vi "LEP_RV_ParseSerialTextOutput.vi"(7 "Serial text":string) -> (1 "Execution time":string, 2 "Stack high water mark":string, 3 "Heap high water mark":string)   [LabVIEW 2011]
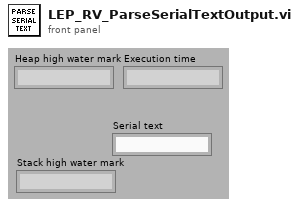
[diagram p1: front panel]
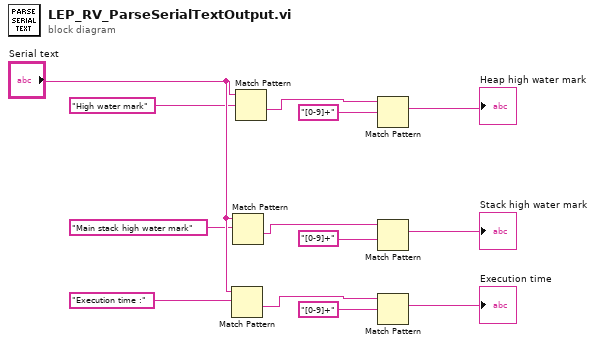
[diagram p0: block diagram]
diagram:
  n1 = Match Pattern(string="Serial text", regular expression="Execution time :") -> (after substring=w3:string)  [unwired: 1 in, 3 out]
  n2 = Match Pattern(string="Serial text", regular expression="Main stack high water mark") -> (after substring=w5:string)  [unwired: 1 in, 3 out]
  n3 = Match Pattern(string="Serial text", regular expression="High water mark") -> (after substring=w4:string)  [unwired: 1 in, 3 out]
  n4 = Match Pattern(string=w4, regular expression="[0-9]+") -> (match substring=→"Heap high water mark":string)  [unwired: 1 in, 3 out]
  n5 = Match Pattern(string=w5, regular expression="[0-9]+") -> (match substring=→"Stack high water mark":string)  [unwired: 1 in, 3 out]
  n6 = Match Pattern(string=w3, regular expression="[0-9]+") -> (match substring=→"Execution time":string)  [unwired: 1 in, 3 out]
